vi "XLP80_Datalog_ConvertDataToString.vi"(8 "error in":errorcluster) -> (0 "error OUT":errorcluster caption="error out", 3 "DataString":string)   [LabVIEW 2021]
uses:
  XLP80_FGlob/1886_FGlob_TDefs_Enum_FGlobItems.ctl
  XLP80_Globals/XLP80_Globals_Status.vi
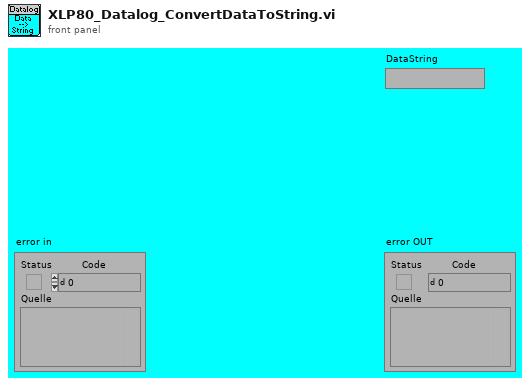
[diagram p1: front panel]
types:
  T1 = typedef "1886_FGlob_TDefs_Enum_FGlobItems.ctl" = enum16{"Put one", "Put all", "Recall one", "Recall all"}
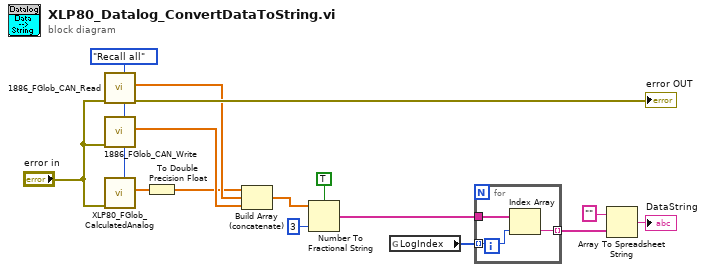
[diagram p0: block diagram]
diagram:
  w4 = 1886_FGlob_TDefs_Enum_FGlobItems."Recall all" ("Function (Recall One)")
  n1 = call "1886_FGlob_CAN_Read.vi"("Function (Recall One)"=w4, "err in"="error in") -> ("err out"=→"error OUT":errorcluster, "AI Values OUT"=w5:dbl[])  [unwired: 7 in, 1 out]
  n2 = call "1886_FGlob_CAN_Write.vi"("Function (Recall One)"=w4, "err in"="error in") -> ("AO Values OUT"=w9:dbl[])  [unwired: 7 in, 2 out]
  n3 = call "XLP80_FGlob_CalculatedAnalog.vi"("Function (Recall One)"=w4, "err in"="error in") -> ("Calc Values OUT"=w3:sgl[])  [unwired: 7 in, 2 out]
  n4 = To Double Precision Float(number=w3) -> (double precision float=w2:dbl[])
  n5 = Build Array (concatenate)(w2, w5, w9) -> (w13:dbl[])
  n6 = Number To Fractional String(use system decimal point (T)=TRUE, number=w13, precision (6)=i16 3) -> (F-format string=w8:string[])  [unwired: 1 in]
  n7 = global read "XLP80_Globals_Status.vi" "LogIndex"() -> (w1:i32[])
  n8 = for {
    tunnel: w1 -> [w17] mode=indexing
    tunnel: w8 -> [w18]
    tunnel: [w16] -> w10 mode=indexing
    n9 = Index Array(array=w18, index=w17) -> (element=w16:string)
  }
  n10 = Array To Spreadsheet String(array=w10, 3:"" ("format string")) -> (spreadsheet string=→"DataString":string)  [unwired: 1 in]
